vi "Highlight.vi"(10 "Field (Panel)":string, 11 "ColumnPanel in":refnum<class "ColumnPanel.lvclass">) -> ()   [LabVIEW 2020, in "Conditum-Tools.lvlib" / "ColumnPanel.lvclass"]
uses:
  ColumnPanel.lvclass
  ColumnPanel.lvclass/ColumnPanel.ctl
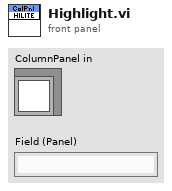
[diagram p1: front panel]
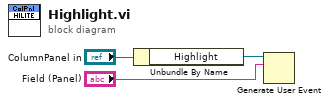
[diagram p0: block diagram]
diagram:
  n1 = Unbundle By Name("ColumnPanel in") -> ("Highlight"=w2:refnum<user-event>)
  n2 = Generate User Event(user event=w2, event data cluster="Field (Panel)") -> ()  [unwired: 2 in, 2 out]
